vi "Prepare Data.vi"(0 "CS in":refnum<class "QCS.lvclass">, 2 "I0":T1 {"Current" min=0.0}, 3 "I1":T1 {"Current" min=0.0}, 4 "I2":T1 {"Current" min=0.0}, 5 "I3":T1 {"Current" min=0.0}, 7 "error in (no error)":errorcluster) -> (18 "Range bits":u32, 20 "CS out":refnum<class "QCS.lvclass">, 21 "V Out 0":dbl, 23 "V Out 1":dbl, 24 "V Out 2":dbl, 25 "V Out 3":dbl, 27 "error out":errorcluster)   [LabVIEW 2016, in "QCS.lvclass"]
uses:
  Lib.llb/QCS.lvclass
  Lib.llb/CS Data.ctl
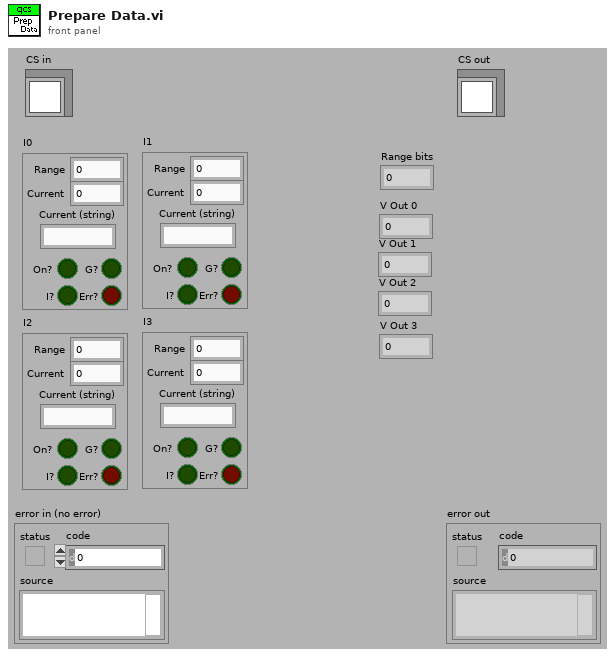
[diagram p1: front panel]
types:
  T1 = typedef "CS Data.ctl" = cluster{"Range":u8, "Current":dbl, "Current (string)":string, "On?":bool, "G?":bool, "I?":bool, "Err?":bool}
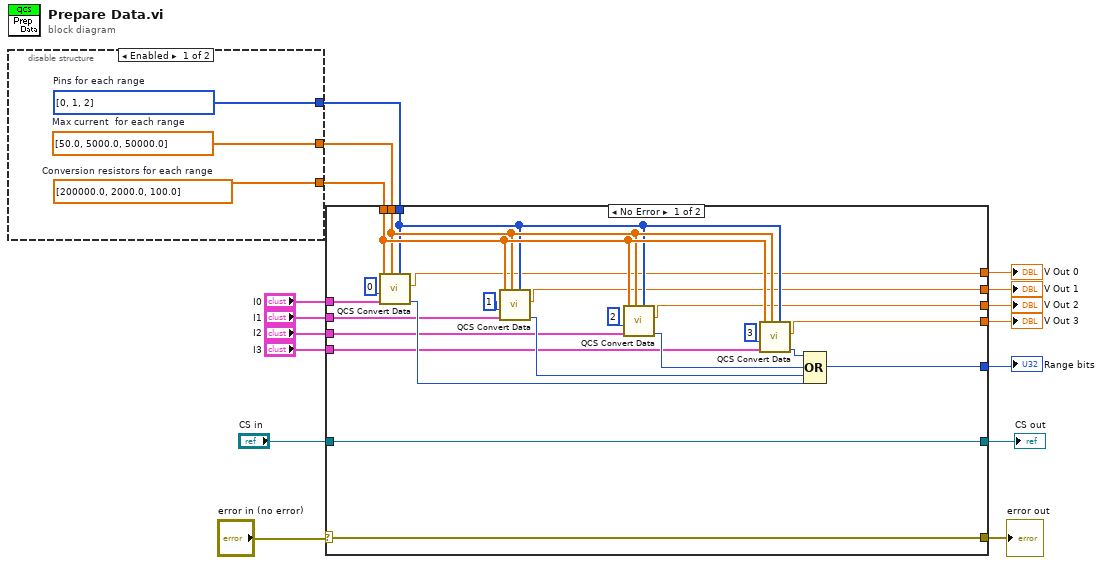
[diagram p0: block diagram]
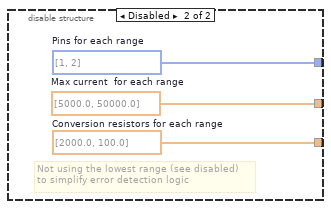
[diagram p2: hidden frame]
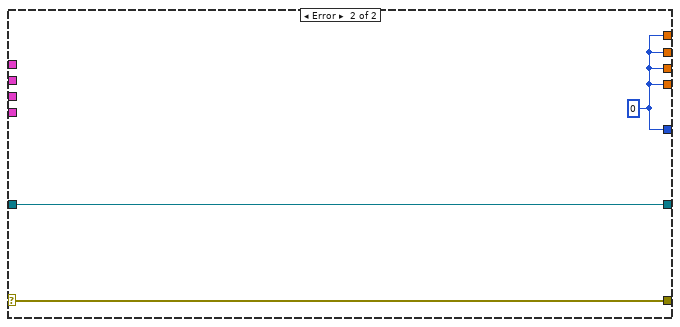
[diagram p3: hidden frame]
diagram:
  n1 = disable-structure shown="Enabled" {
    disable-tunnel: [w19 w22] -> w10
    disable-tunnel: [w18 w21] -> w9
    disable-tunnel: [w17 w20] -> w8
    frame Enabled {
      w19 = dbl[] [200000.0, 2000.0, 100.0]  # Conversion resistors for each range
      w17 = u8[] [0, 1, 2]  # Pins for each range
      w18 = dbl[] [50.0, 5000.0, 50000.0]  # Max current  for each range
    }
    frame Disabled {
      w20 = u8[] [1, 2]  # Pins for each range
      w21 = dbl[] [5000.0, 50000.0]  # Max current  for each range
      w22 = dbl[] [2000.0, 100.0]  # Conversion resistors for each range
      # "Not using the lowest range (see disabled)\nto simplify error detection logic"
    }
  }
  n2 = case shown="No Error" "error in (no error)" {
    selector: "error in (no error)" -> [w28 w47]
    tunnel: [w28 w47] -> w15
    tunnel: "I0" -> [w30 _]
    tunnel: "I1" -> [w31 _]
    tunnel: "I2" -> [w32 _]
    tunnel: "I3" -> [w33 _]
    tunnel: w10 -> [w40 _]
    tunnel: w9 -> [w35 _]
    tunnel: w8 -> [w34 _]
    tunnel: [w29 w46] -> w7
    tunnel: [w27 w46] -> w3
    tunnel: [w26 w46] -> w4
    tunnel: [w25 w46] -> w5
    tunnel: [w24 w46] -> w6
    tunnel: "CS in" -> [w23 w45]
    tunnel: [w23 w45] -> w1
    frame No Error {
      n3 = call "QCS Convert Data.vi"("Pins for each range"=w34, "Max current for each range"=w35, "I In"=w30, "Channel"=0, "Conversion resistors for each range"=w40) -> ("Range Bits"=w36:u32, "V Out"=w24:dbl)  [unwired: 3 in]
      n4 = call "QCS Convert Data.vi"("Pins for each range"=w34, "Max current for each range"=w35, "I In"=w31, "Channel"=1, "Conversion resistors for each range"=w40) -> ("Range Bits"=w37:u32, "V Out"=w25:dbl)  [unwired: 3 in]
      n5 = call "QCS Convert Data.vi"("Pins for each range"=w34, "Max current for each range"=w35, "I In"=w32, "Channel"=2, "Conversion resistors for each range"=w40) -> ("Range Bits"=w38:u32, "V Out"=w26:dbl)  [unwired: 3 in]
      n6 = call "QCS Convert Data.vi"("Pins for each range"=w34, "Max current for each range"=w35, "I In"=w33, "Channel"=3, "Conversion resistors for each range"=w40) -> ("Range Bits"=w39:u32, "V Out"=w27:dbl)  [unwired: 3 in]
      n7 = Compound Arithmetic op=OR(w39, w38, w37, w36) -> (w29:u32)
    }
    frame Error {
      w46 = u32 0
    }
  }
  "error out" <- w15
  "Range bits" <- w7
  "V Out 0" <- w6
  "V Out 1" <- w5
  "V Out 2" <- w4
  "V Out 3" <- w3
  "CS out" <- w1
